vi "test_DeviceManager_OpenWebSocketCommunication.vi"(8 "error in":errorcluster) -> (0 "error out":errorcluster, 3 "Pass":bool)   [LabVIEW 2023]
doc: "_____\nCreated using DQMH Event Scripter 7.0.0.1280."
uses:
  Source/Libraries/DeviceManager/DeviceManager.lvlib
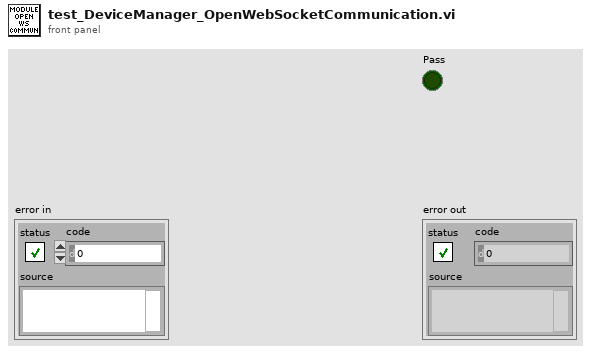
[diagram p1: front panel]
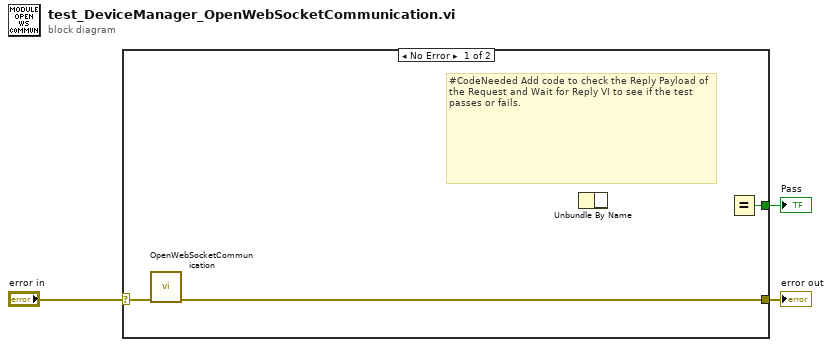
[diagram p0: block diagram]
diagram:
  n1 = case shown="No Error" "error in" {
    selector: "error in" -> [w6 w7]
    tunnel: [w5 w7] -> w2
    tunnel: [w4 _] -> w1
    frame No Error {
      # "#CodeNeeded Add code to check the Reply Payload of the Request and Wait for Reply VI to see if the test passes or fails."
      n2 = call "OpenWebSocketCommunication.vi"("error in"=w6) -> ("error out"=w5:errorcluster)  [unwired: 8 in, 2 out]
      n3 = Unbundle By Name() -> ()  [unwired: 1 in, 1 out]
      n4 = Equal?() -> (x = y?=w4:bool)  [unwired: 2 in]
    }
    frame Error {
    }
  }
  "error out" <- w2
  "Pass" <- w1
